vi "Change Color.vi"(8 "error in (no error)":errorcluster, 10 "Command":enum16{"Normal", "Alarm", "Bypass", "Tamper"}[](array[ring]), 11 "AllObjs[]":refnum<vi>[](array[refnum])) -> (0 "error out":errorcluster)   [LabVIEW 2013]
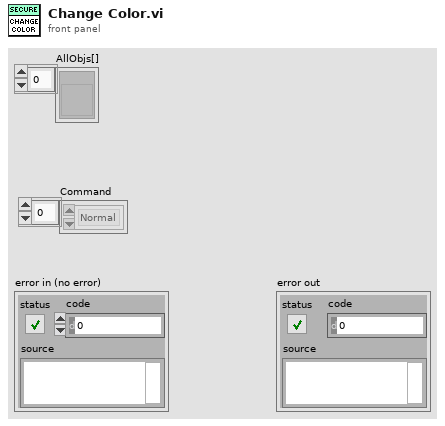
[diagram p1: front panel]
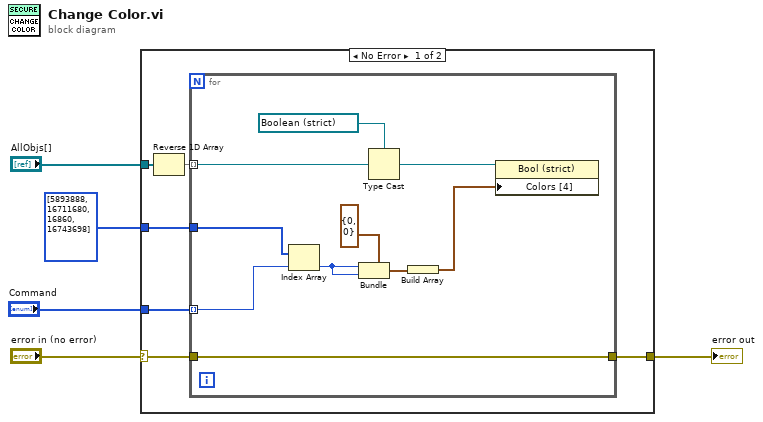
[diagram p0: block diagram]
diagram:
  n1 = case shown="No Error" "error in (no error)" {
    selector: "error in (no error)" -> [w7 w22]
    tunnel: "AllObjs[]" -> [w11 _]
    tunnel: "Command" -> [w10 _]
    tunnel: [w8 w22] -> w5
    tunnel: u32[] [5893888, 16711680, 16860, 16743698] -> [w6 _]
    frame No Error {
      n2 = Reverse 1D Array(array=w11) -> (reversed array=w9:refnum<vi>[])
      n3 = for {
        tunnel: w10 -> [w21] mode=indexing
        tunnel: w9 -> [w20] mode=indexing
        tunnel: [w13] -> w8
        tunnel: w7 -> [w13]
        tunnel: w6 -> [w12]
        n4 = Index Array(array=w12, index=w21) -> (element=w16:u32)
        n5 = Bundle(cluster=cluster{u32, u32} {0, 0}, w16, w16) -> (w15:cluster{u32, u32})
        n6 = Type Cast(type=refnum<vi> refnum ("reference"), x=w20) -> (*(type *) &x=w19:refnum<vi>)
        n7 = Build Array(w15) -> (w14:cluster{u32, u32}[])
        n8 = property on="Property Node" class="Bool (strict)"(reference=w19, "Colors [4]"=w14) -> ()  [unwired: 1 in, 2 out]
      }
    }
    frame Error {
    }
  }
  "error out" <- w5
